vi "Commands to ITX.vi"(1 "Commands":string) -> (0 "ITX Commands":string)   [LabVIEW 2016, in "LV to ITX.lvclass"]
uses:
  LV to ITX.lvclass
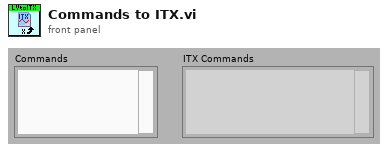
[diagram p1: front panel]
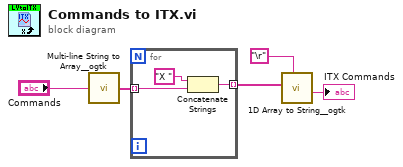
[diagram p0: block diagram]
diagram:
  n1 = call <userlib>:"Multi-line String to Array__ogtk.vi"("string"="Commands") -> ("lines"=w3:string[])
  n2 = for {
    tunnel: w3 -> [w7] mode=indexing
    tunnel: [w6] -> w2 mode=indexing
    n3 = Concatenate Strings("X " ("string"), w7) -> (w6:string)
  }
  n4 = call <userlib>:"1D Array to String__ogtk.vi"("delimiter (Tab)"="\r", "Array of Strings"=w2) -> ("delimited string"=→"ITX Commands":string)  [unwired: 9 in]
